vi "Day 11 - Cosmic Expansion.vi"() -> ()   [LabVIEW 2020, in "AoC 2023.lvlib"]
uses:
  AoC 2023.lvlib
  1460cd73-e12a-485b-9d7d-8782a7466a04.vi
  2c12147c-fff0-40a0-a29f-26f4e772627b.vi
  42862fd3-dd1f-4cee-9aa8-5d502f721ab8.vi
  5916b52d-a21f-453d-9ab9-da4a37886fe3.vi
  2c12147c-fff0-40a0-a29f-26f4e772627b.vi/35b1f6c1-b35f-44f2-9ba0-5546a8eaac0a.vi
  5916b52d-a21f-453d-9ab9-da4a37886fe3.vi/35b1f6c1-b35f-44f2-9ba0-5546a8eaac0a.vi
panel:
  in  "Expansion Rate":i32=1000000
  in  "Tab Control":enum32{"GRID"}(tab)
  out "GRID":string[][](array[string])
  in  "TIMEOUT":i32
  out "Puzzle Part-2 Answer":string
  out "Puzzle Answer":string
  in  "Puzzle Inputs":string[](array[string])=["...#......\n.......#..\n#.........\n..........\n......#...\n.#........\n.........#\n..........\n.......#..\n#...#....."]
  # "Enter the Puzzle Input and run the VI"
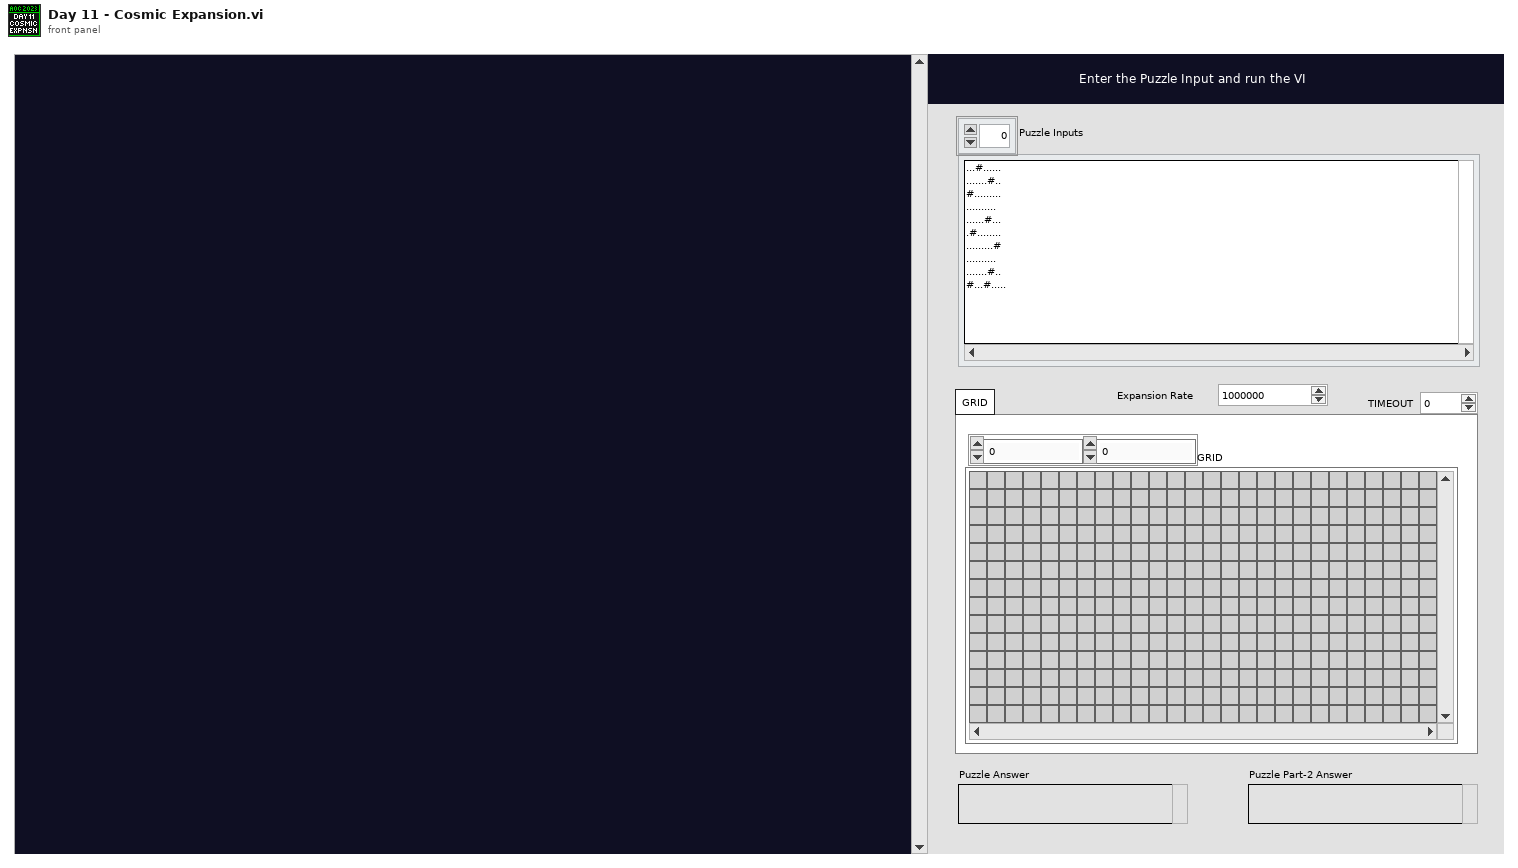
[diagram p1: front panel]
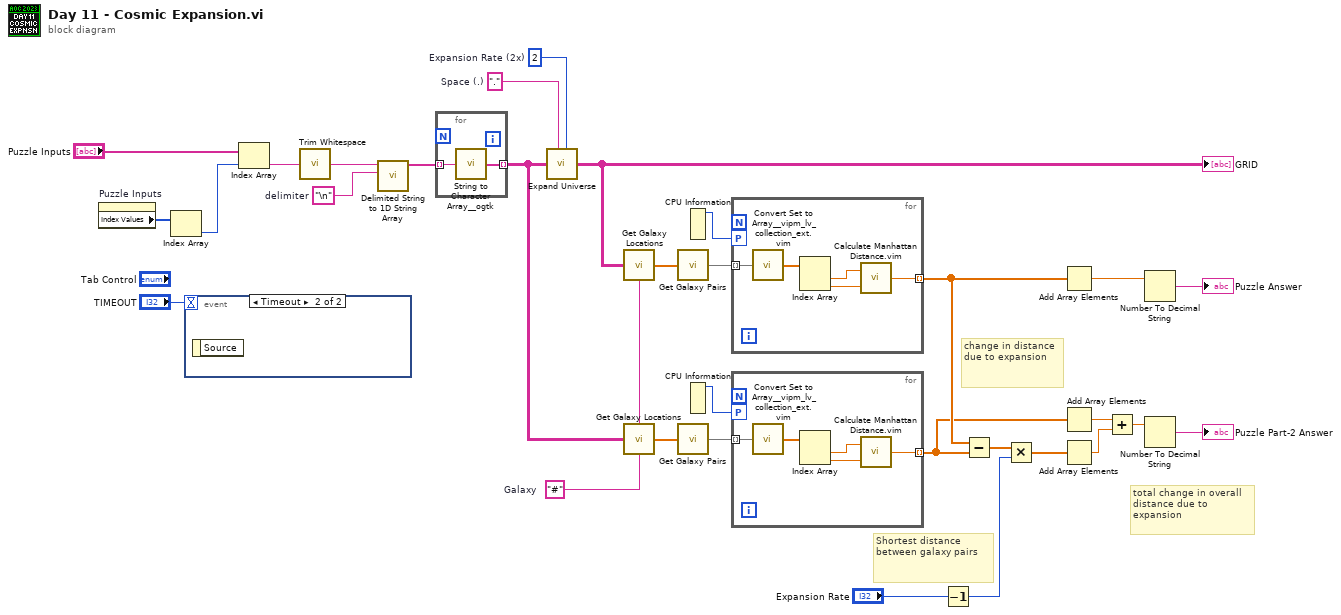
[diagram p0: block diagram]
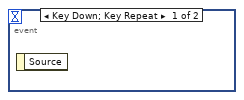
[diagram p2: hidden frame]
diagram:
  w17 = 2  # Expansion Rate (2x)
  w13 = "#"  # Galaxy
  w14 = "."  # Space (.)
  w29 = "\n"  # delimiter
  # "total change in overall distance due to expansion"
  # "change in distance due to expansion"
  # "Shortest distance between galaxy pairs"
  n1 = property on="Puzzle Inputs" class="Arr (strict)"() -> ("Index Values"=w24:u32[])  [unwired: 2 in, 2 out]
  n2 = Index Array(array=w24) -> (element=w23:u32)  [unwired: 1 in]
  n3 = event shown="[1] Timeout" {
    selector: _ -> [_ _]
    dyn-events: _ -> [_ _]
    timeout: "TIMEOUT" -> [_ _]
    event Key Down; Key Repeat {
      n4 = event-data() -> ()  [unwired: 1 in, 1 out]
    }
    event Timeout {
      n5 = event-data() -> ()  [unwired: 1 in, 1 out]
    }
  }
  n6 = Index Array(array="Puzzle Inputs", index=w23) -> (element=w25:string)
  n7 = call <vilib>:"Trim Whitespace.vi"("string"=w25) -> ("trimmed string"=w28:string)  [unwired: 1 in]
  n8 = call <vilib>:"Delimited String to 1D String Array.vi"("delimiter"=w29, "delimited string"=w28) -> ("string array"=w27:string[])  [unwired: 9 in]
  n9 = for {
    tunnel: w27 -> [w33] mode=indexing
    tunnel: [w32] -> w15 mode=indexing
    n10 = call <userlib>:"String to Character Array__ogtk.vi"("Input String"=w33) -> ("Character Array"=w32:string[])
  }
  n11 = call "Expand Universe.vi"("Universe"=w15, "Space (.)"=w14, "Expansion Rate (2x)"=w17) -> ("Expanded Universe"=w21:string[][])
  "GRID" <- w21
  n12 = call "Get Galaxy Locations.vi"("Universe"=w21, "Galaxy (#)"=w13) -> ("Galaxy Locations"=w20:cdb[])
  n13 = call "Get Galaxy Locations.vi"("Universe"=w15, "Galaxy (#)"=w13) -> ("Galaxy Locations"=w10:cdb[])
  n14 = call "Get Galaxy Pairs.vi"("Galaxy Locations"=w20) -> ("Galaxy Pairs"=w19:set{set{cdb}})  [unwired: 1 in]
  n15 = call "Get Galaxy Pairs.vi"("Galaxy Locations"=w10) -> ("Galaxy Pairs"=w11:set{set{cdb}})  [unwired: 1 in]
  n16 = CPU Information() -> (4:w16:i32)  [unwired: 3 out]
  n17 = CPU Information() -> (4:w12:i32)  [unwired: 3 out]
  n18 = for {
    tunnel: w19 -> [w35] mode=indexing
    tunnel: [w34] -> w9 mode=indexing
    workers-P: w16 -> [_]
    n19 = call "Convert Set to Array__vipm_lv_collection_ext.vim"("set"=w35) -> ("array"=w38:cdb[])  [unwired: 8 in]
    n20 = Index Array(array=w38) -> (element #1=w37:cdb, element #2=w36:cdb)  [unwired: 2 in]
    n21 = call "Calculate Manhattan Distance.vim"("Location 2"=w36, "Location 1"=w37) -> ("Manhatten Distance"=w34:dbl)
  }
  n22 = for {
    tunnel: w11 -> [w40] mode=indexing
    tunnel: [w39] -> w3 mode=indexing
    workers-P: w12 -> [_]
    n23 = call "Convert Set to Array__vipm_lv_collection_ext.vim"("set"=w40) -> ("array"=w43:cdb[])  [unwired: 8 in]
    n24 = Index Array(array=w43) -> (element #1=w42:cdb, element #2=w41:cdb)  [unwired: 2 in]
    n25 = call "Calculate Manhattan Distance.vim"("Location 2"=w41, "Location 1"=w42) -> ("Manhatten Distance"=w39:dbl)
  }
  n26 = Decrement(x="Expansion Rate") -> (x-1=w1:i32)
  n27 = Subtract(x=w9, y=w3) -> (x-y=w7:dbl[])
  n28 = Multiply(x=w7, y=w1) -> (x*y=w8:dbl[])
  n29 = Add Array Elements(numeric array=w9) -> (sum=w18:dbl)
  n30 = Add Array Elements(numeric array=w3) -> (sum=w6:dbl)
  n31 = Add Array Elements(numeric array=w8) -> (sum=w5:dbl)
  n32 = Add(x=w6, y=w5) -> (x+y=w4:dbl)
  n33 = Number To Decimal String(number=w18) -> (decimal integer string=→"Puzzle Answer":string)  [unwired: 1 in]
  n34 = Number To Decimal String(number=w4) -> (decimal integer string=→"Puzzle Part-2 Answer":string)  [unwired: 1 in]
